vi "DC_CNTRL_start_up.vi"(0 "Device Index":u32, 1 "Box Number":u16(ring) items=["1", "2"], 3 "Input Potentials":dbl[](array[numeric]), 11 "error in (no error)":errorcluster) -> (4 "Handle out":u64, 12 "Device Information":T1 {"Type" items=["FT232B-FT245B", "FT8U232AM-FT8U245AM", "FT8U100AX", "UNKNOWN", "FT2232", "FT232R-FT245R", "FT2232H", "FT4232H", "FT232H"]}, 14 "Max Range Array":dbl[](array[numeric]), 15 "error out":errorcluster)   [LabVIEW 2019]
uses:
  <vilib>/Utility/config.llb/Write Key (Double).vi
  <vilib>/Utility/config.llb/Read Key (Double).vi
  <vilib>/Utility/config.llb/NI_LVConfig.lvlib
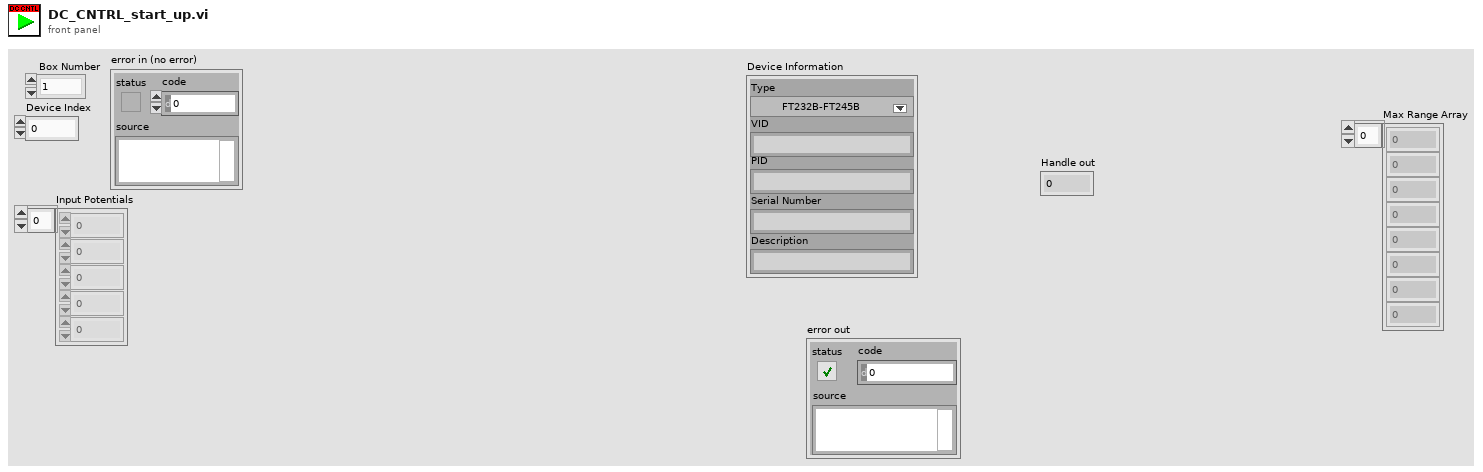
[diagram p1: front panel]
types:
  T1 = cluster{"Type":u32, "VID":string, "PID":string, "Serial Number":string, "Description":string}
  T2 = typedef "NI_LVConfig.lvlib/Config Data RefNum.ctl" = refnum<k1>
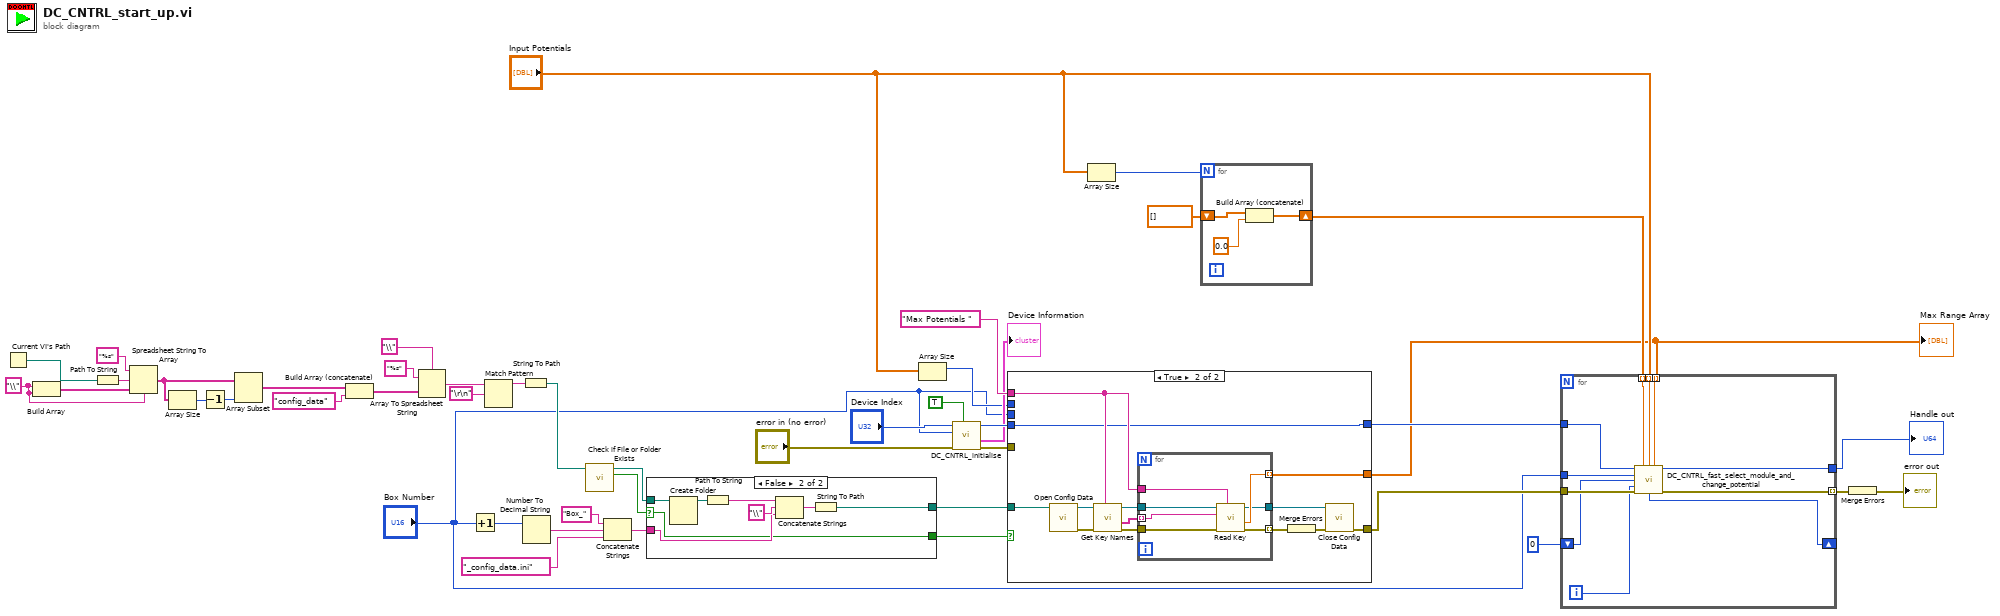
[diagram p0: block diagram]
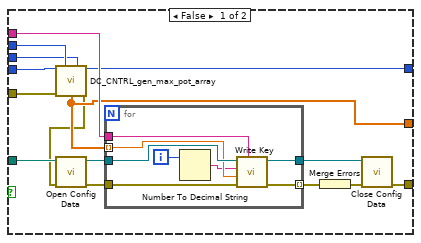
[diagram p2: hidden frame]
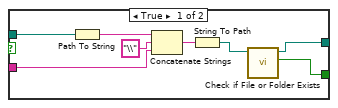
[diagram p3: hidden frame]
diagram:
  w44 = "\\" ("delimiter (Tab)")
  n1 = Current VI's Path() -> (path=w46:path)
  n2 = Build Array(w44, w44) -> (w43:string[])
  n3 = Path To String(path=w46) -> (string=w45:string)
  n4 = Spreadsheet String To Array(delimiter (Tab)=w44, format string="%s", spreadsheet string=w45, array type (2D Dbl)=w43) -> (array=w41:string[])
  n5 = Array Size(array=w41) -> (size(s)=w37:i32)
  n6 = Decrement(x=w37) -> (x-1=w40:i32)
  n7 = Array Subset(array=w41, length=w40) -> (w36:string[])  [unwired: 1 in]
  n8 = Build Array (concatenate)(w36, "config_data") -> (w34:string[])
  n9 = Array To Spreadsheet String(delimiter (Tab)="\\", array=w34, 3:"%s" ("format string")) -> (spreadsheet string=w32:string)
  n10 = Increment(x="Box Number") -> (x+1=w28:u16)
  n11 = Match Pattern(string=w32, regular expression="\r\n") -> (before substring=w31:string)  [unwired: 1 in, 3 out]
  n12 = String To Path(string=w31) -> (path=w33:path)
  n13 = Number To Decimal String(number=w28) -> (decimal integer string=w26:string)  [unwired: 1 in]
  n14 = call <vilib>:"Check if File or Folder Exists.vi"("path"=w33) -> ("file or folder exists?"=w29:bool, "dup path"=w24:path)  [unwired: 8 in, 1 out]
  n15 = Concatenate Strings("Box_", w26, "_config_data.ini") -> (w23:string)
  n16 = case shown="False" w29 {
    selector: w29 -> [_ w57]
    tunnel: w24 -> [w50 w56]
    tunnel: w23 -> [w52 w60]
    tunnel: [w47 w58] -> w21
    tunnel: [w48 w57] -> w22
    frame True {
      n17 = Path To String(path=w50) -> (string=w54:string)
      n18 = Concatenate Strings(w54, "\\" ("element"), w52) -> (w51:string)
      n19 = String To Path(string=w51) -> (path=w49:path)
      n20 = call <vilib>:"Check if File or Folder Exists.vi"("path"=w49) -> ("file or folder exists?"=w48:bool, "dup path"=w47:path)  [unwired: 8 in, 1 out]
    }
    frame False {
      n21 = Create Folder(path (use dialog)=w56) -> (created path=w55:path)  [unwired: 2 in, 2 out]
      n22 = Path To String(path=w55) -> (string=w62:string)
      n23 = Concatenate Strings(w62, "\\" ("element"), w60) -> (w59:string)
      n24 = String To Path(string=w59) -> (path=w58:path)
    }
  }
  n25 = Array Size(array="Input Potentials") -> (size(s)=w13:i32)
  n26 = call "DC_CNTRL_initialise.vi"("Check status?"=TRUE, "error in (no error)"="error in (no error)", "Box Number"="Box Number", "Device Index"="Device Index") -> ("error out"=w18:errorcluster, "Device Information"=→"Device Information":T1, "Handle out"=w19:u64)  [unwired: 5 in]
  n27 = case shown="True" w22 {
    tunnel: w21 -> [w77 w98]
    tunnel: [w71 w91] -> w12
    tunnel: "Max Potentials " ("section") -> [w70 w90]
    tunnel: [w69 w88] -> w6
    tunnel: w19 -> [w68 w86]
    tunnel: w18 -> [w67 _]
    tunnel: [w66 w86] -> w11
    tunnel: w13 -> [w65 _]
    tunnel: "Box Number" -> [w64 _]
    frame False {
      n28 = call "DC_CNTRL_gen_max_pot_array.vi"("Handle"=w68, "Number of supplies in box"=w65, "Box Number"=w64, "error in (no error)"=w67) -> ("Handle out"=w66:u64, "Max Range Aray"=w69:dbl[], "error out"=w63:errorcluster)  [unwired: 9 in]
      n29 = call <vilib>:"Open Config Data.vi"("error in (no error)"=w63, "configuration file path"=w77) -> ("error out"=w75:errorcluster, "refnum"=w76:T2)  [unwired: 7 in, 1 out]
      n30 = for {
        tunnel: w69 -> [w81] mode=indexing
        tunnel: w76 -> [w85]
        tunnel: w75 -> [w84]
        tunnel: [w83] -> w74
        tunnel: [w82] -> w73 mode=indexing
        tunnel: w70 -> [w78]
        i -> [w80]
        n31 = Number To Decimal String(number=w80) -> (decimal integer string=w79:string)  [unwired: 1 in]
        n32 = call-poly <vilib>:"Write Key.vi"("section"=w78, "error in (no error)"=w84, "value"=w81, "key"=w79, "refnum"=w85) -> ("error out"=w82:errorcluster, "refnum out"=w83:T2)  [unwired: 4 in, 1 out]
      }
      n33 = Merge Errors(w73) -> (w72:errorcluster)
      n34 = call <vilib>:"Close Config Data.vi"("error in (no error)"=w72, "refnum"=w74) -> ("error out"=w71:errorcluster)  [unwired: 8 in, 1 out]
    }
    frame True {
      n35 = call <vilib>:"Open Config Data.vi"("configuration file path"=w98) -> ("error out"=w96:errorcluster, "refnum"=w97:T2)  [unwired: 8 in, 1 out]
      n36 = call <vilib>:"Get Key Names.vi"("section"=w90, "error in (no error)"=w96, "refnum"=w97) -> ("error out"=w94:errorcluster, "key names"=w95:string[], "refnum out"=w87:T2)  [unwired: 5 in, 1 out]
      n37 = for {
        tunnel: w95 -> [w105] mode=indexing
        tunnel: w94 -> [w104]
        tunnel: [w103] -> w93 mode=indexing
        tunnel: [w102] -> w88 mode=indexing
        tunnel: w90 -> [w101]
        tunnel: [w100] -> w89
        tunnel: w87 -> [w99]
        n38 = call-poly <vilib>:"Read Key.vi"("section"=w101, "error in (no error)"=w104, "key"=w105, "refnum"=w99) -> ("error out"=w103:errorcluster, "value"=w102:dbl, "refnum out"=w100:T2)  [unwired: 4 in, 1 out]
      }
      n39 = Merge Errors(w93) -> (w92:errorcluster)
      n40 = call <vilib>:"Close Config Data.vi"("error in (no error)"=w92, "refnum"=w89) -> ("error out"=w91:errorcluster)  [unwired: 8 in, 1 out]
    }
  }
  "Max Range Array" <- w6
  n41 = Array Size(array="Input Potentials") -> (size(s)=w9:i32)
  n42 = for {
    N: w9 -> [_]
    shift-right: [w106] -> w7
    shift-left: dbl[] [] -> [w107]
    n43 = Build Array (concatenate)(w107, 0.0 ("element")) -> (w106:dbl[])
  }
  n44 = for {
    tunnel: w12 -> [w119]
    tunnel: w11 -> [w118]
    tunnel: "Input Potentials" -> [w117] mode=indexing
    tunnel: w7 -> [w116] mode=indexing
    tunnel: w6 -> [w115] mode=indexing
    shift-right: [w111] -> _
    shift-left: 0 -> [w113]
    tunnel: "Box Number" -> [w112]
    tunnel: [w110] -> w3 mode=indexing
    tunnel: [w109] -> w1
    i -> [w114]
    n45 = call "DC_CNTRL_fast_select_module_and_change_potential.vi"("Handle"=w118, "Current Potential (V)"=w116, "Target Potential (V)"=w117, "Max Potential (V)"=w115, "Box Number"=w112, "Current Module Number"=w113, "Desired Module Number"=w114, "error in (no error)"=w119) -> ("Handle out"=w109:u64, "Current Module Number Out"=w111:u16, "error out"=w110:errorcluster)  [unwired: 5 in]
  }
  "Handle out" <- w1
  n46 = Merge Errors(w3) -> (→"error out":errorcluster)
